vi "Main.vi"() -> ()   [LabVIEW 2020]
uses:
  <vilib>/Utility/NIReport.llb/Create Report.vi
  <vilib>/addons/_office/excel.llb/Excel Get Data.vi
  <vilib>/addons/_office/excel.llb/Excel Get Data ([str]).vi
  <vilib>/Utility/NIReport.llb/NI_report.lvclass
panel:
  in  "文件路径":path
  out "计时器":i32 caption="已用时间(s)" format="%<%H:%M:%S>t"
  in  "过程停止按钮":bool
  in  "复位按钮":bool
  out "结束指示灯":bool
  out "数据导入指示灯":bool
  out "显示屏":string
  in  "抽取按钮":bool
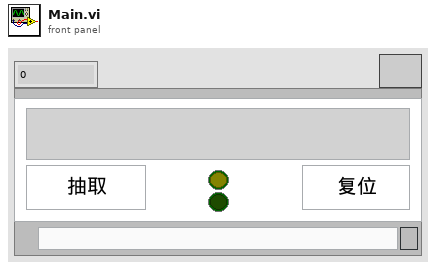
[diagram p1: front panel]
types:
  T1 = enum8{"Enabled", "Disabled", "Disabled and Grayed Out"}
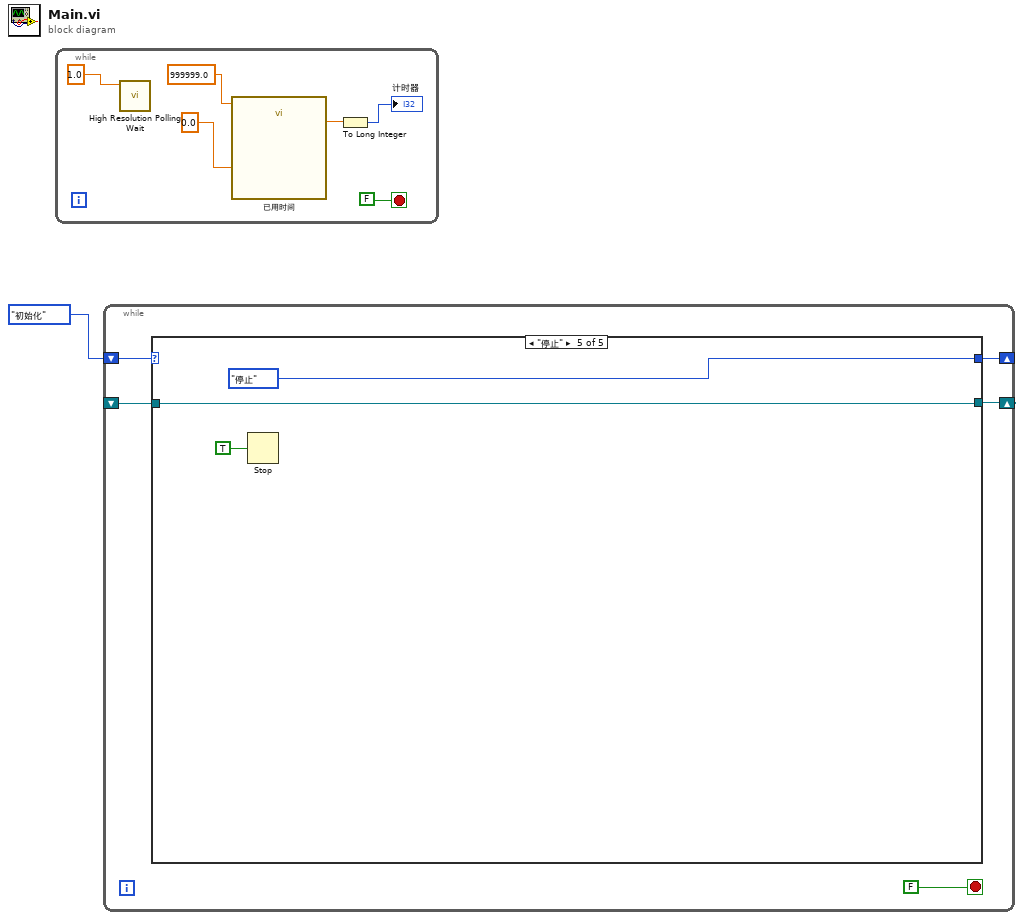
[diagram p0: block diagram]
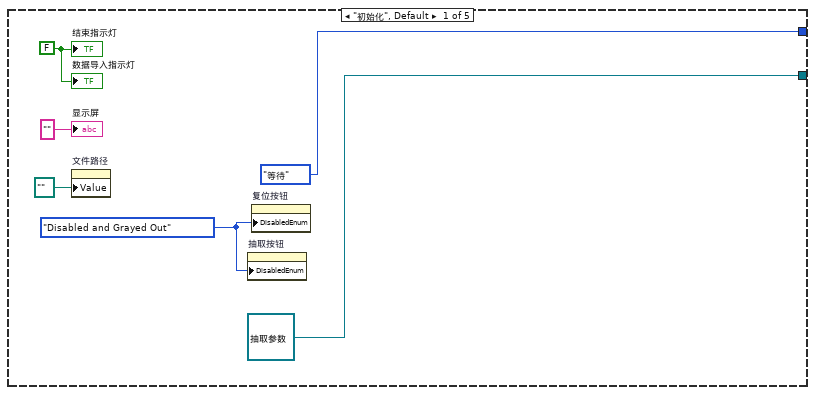
[diagram p2: hidden frame]
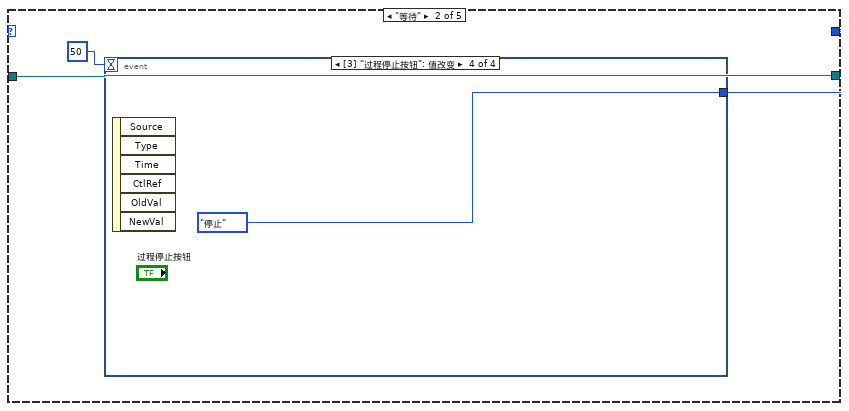
[diagram p3: hidden frame]
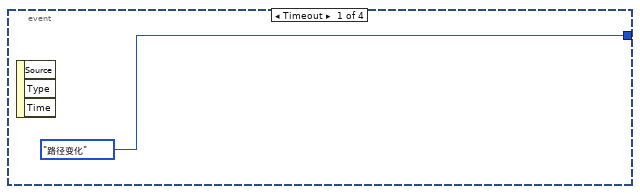
[diagram p4: hidden frame]
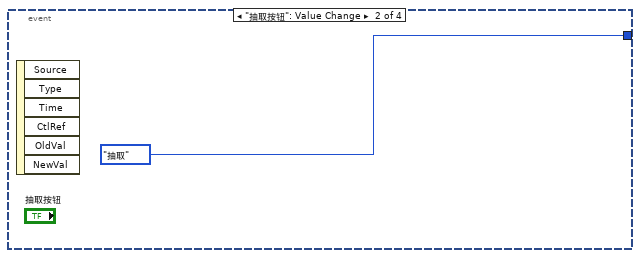
[diagram p5: hidden frame]
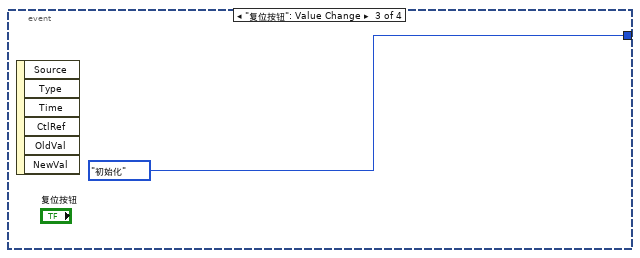
[diagram p6: hidden frame]
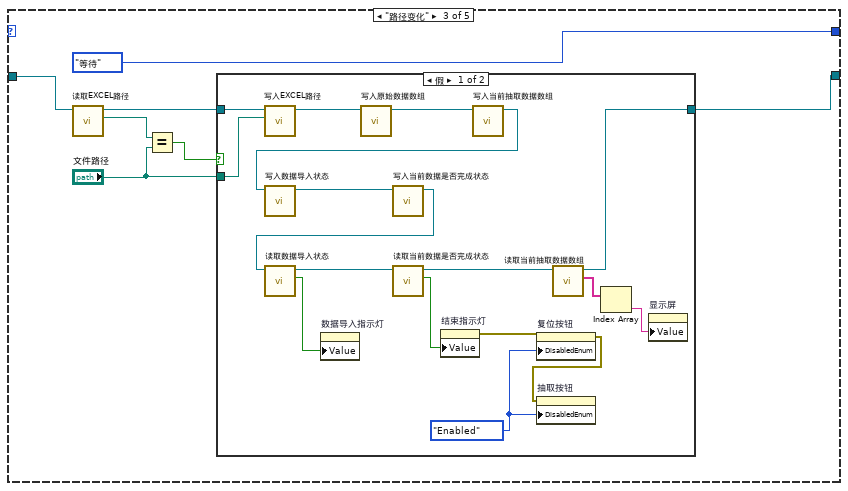
[diagram p7: hidden frame]
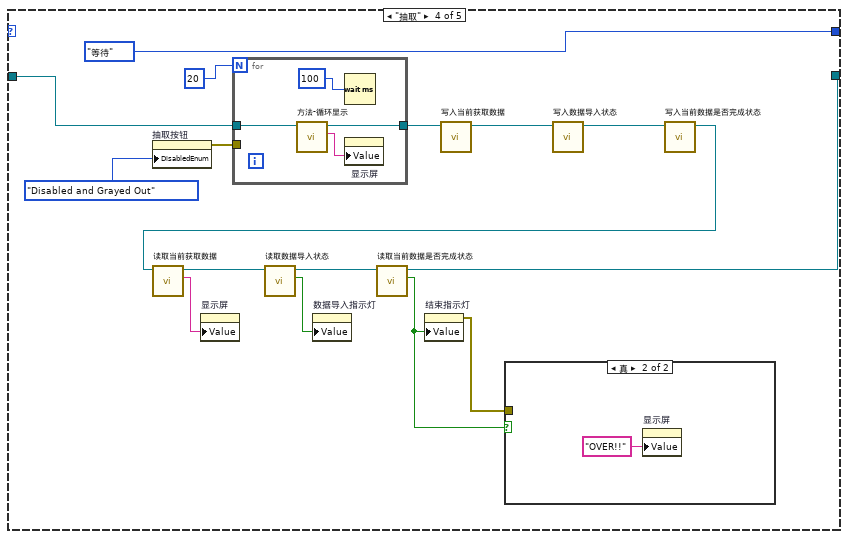
[diagram p9: hidden frame]
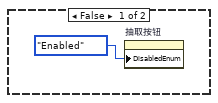
[diagram p10: hidden frame]
diagram:
  n1 = while {
    stop <- FALSE stop-if-true
    n2 = call <vilib>:"High Resolution Polling Wait.vi"("seconds to wait"=1.0) -> ()  [unwired: 10 in, 1 out]
    n3 = call "已用时间"("Time Target (s)"=999999.0, "Set Start Time (s)"=0.0) -> ("Elapsed Time (s)"=w4:dbl)  [unwired: 10 in, 7 out]
    n4 = To Long Integer(number=w4) -> (32bit integer=→"计时器":i32)
  }
  n5 = while {
    shift-right: [w11] -> _
    shift-left: enum16{"初始化", "等待", "路径变化", "抽取", "停止"}."初始化" -> [w12]
    shift-right: [w10] -> _
    shift-left: _ -> [w9]
    stop <- FALSE stop-if-true
    n6 = case shown="\"停止\"" w12 {
      tunnel: [enum16{"初始化", "等待", "路径变化", "抽取", "停止"}."等待" w20 enum16{"初始化", "等待", "路径变化", "抽取", "停止"}."等待" enum16{"初始化", "等待", "路径变化", "抽取", "停止"}."等待" enum16{"初始化", "等待", "路径变化", "抽取", "停止"}."停止"] -> w11
      tunnel: [refnum<class "抽取参数.lvclass"> refnum ("抽取参数.lvclass") w19 w27 w52 w74] -> w10
      tunnel: w9 -> [_ w19 w31 w62 w74]
      frame "初始化", Default {
        w15 = T1."Disabled and Grayed Out" ("禁用")
        w18 = FALSE ("结束指示灯")
        n7 = property on="文件路径" class="Path"("Value"=path "" ("文件路径")) -> ()  [unwired: 2 in, 2 out]
        n8 = property on="抽取按钮" class="Bool"("DisabledEnum"=w15) -> ()  [unwired: 2 in, 2 out]
        n9 = property on="复位按钮" class="Bool"("DisabledEnum"=w15) -> ()  [unwired: 2 in, 2 out]
        "结束指示灯" <- w18
        "数据导入指示灯" <- w18
        "显示屏" <- "" ("显示屏")
      }
      frame "等待" {
        n10 = event shown="[3] \"过程停止按钮\": 值改变" {
          selector: _ -> [_ _ _ _]
          dyn-events: _ -> [_ _ _ _]
          timeout: 50 -> [_ _ _ _]
          tunnel: [enum16{"初始化", "等待", "路径变化", "抽取", "停止"}."路径变化" enum16{"初始化", "等待", "路径变化", "抽取", "停止"}."抽取" enum16{"初始化", "等待", "路径变化", "抽取", "停止"}."初始化" enum16{"初始化", "等待", "路径变化", "抽取", "停止"}."停止"] -> w20
          event Timeout {
            n11 = event-data() -> ()  [unwired: 1 in, 3 out]
          }
          event "抽取按钮": Value Change {
            n12 = event-data() -> ()  [unwired: 1 in, 6 out]
          }
          event "复位按钮": Value Change {
            n13 = event-data() -> ()  [unwired: 1 in, 6 out]
          }
          event "过程停止按钮": Value Change {
            n14 = event-data() -> ()  [unwired: 1 in, 6 out]
          }
        }
      }
      frame "路径变化" {
        n15 = call "读取EXCEL路径.vi"("抽取参数输入"=w31) -> ("EXCEL路径"=w30:path, "抽取参数输出"=w28:refnum<class "抽取参数.lvclass">)  [unwired: 8 in, 1 out]
        n16 = Equal?(x=w30, y="文件路径") -> (x = y?=w29:bool)
        n17 = case shown="假" w29 {
          tunnel: w28 -> [w49 w50]
          tunnel: [w33 w50] -> w27
          tunnel: "文件路径" -> [w48 _]
          frame False {
            w39 = T1."Enabled" ("禁用")
            n18 = call "写入EXCEL路径.vi"("EXCEL路径"=w48, "抽取参数输入"=w49) -> ("抽取参数输出"=w47:refnum<class "抽取参数.lvclass">)  [unwired: 8 in, 1 out]
            n19 = call "写入原始数据数组.vi"("抽取参数输入"=w47) -> ("抽取参数输出"=w46:refnum<class "抽取参数.lvclass">)  [unwired: 9 in, 1 out]
            n20 = call "写入当前抽取数据数组.vi"("抽取参数输入"=w46) -> ("抽取参数输出"=w45:refnum<class "抽取参数.lvclass">)  [unwired: 9 in, 1 out]
            n21 = call "写入数据导入状态.vi"("抽取参数输入"=w45) -> ("抽取参数输出"=w44:refnum<class "抽取参数.lvclass">)  [unwired: 9 in, 1 out]
            n22 = call "写入当前数据是否完成状态.vi"("抽取参数输入"=w44) -> ("抽取参数输出"=w43:refnum<class "抽取参数.lvclass">)  [unwired: 9 in, 1 out]
            n23 = call "读取数据导入状态.vi"("抽取参数输入"=w43) -> ("数据导入状态"=w42:bool, "抽取参数输出"=w41:refnum<class "抽取参数.lvclass">)  [unwired: 8 in, 1 out]
            n24 = property on="数据导入指示灯" class="Bool (严格)"("Value"=w42) -> ()  [unwired: 2 in, 2 out]
            n25 = call "读取当前数据是否完成状态.vi"("抽取参数输入"=w41) -> ("当前数据是否完成状态"=w40:bool, "抽取参数输出"=w36:refnum<class "抽取参数.lvclass">)  [unwired: 8 in, 1 out]
            n26 = property on="结束指示灯" class="Bool (严格)"("Value"=w40) -> (error out=w38:errorcluster)  [unwired: 2 in, 1 out]
            n27 = property on="复位按钮" class="Bool"(error in=w38, "DisabledEnum"=w39) -> (error out=w37:errorcluster)  [unwired: 1 in, 1 out]
            n28 = property on="抽取按钮" class="Bool"(error in=w37, "DisabledEnum"=w39) -> ()  [unwired: 1 in, 2 out]
            n29 = call "读取当前抽取数据数组.vi"("抽取参数输入"=w36) -> ("当前抽取数据数组"=w35:string[], "抽取参数输出"=w33:refnum<class "抽取参数.lvclass">)  [unwired: 8 in, 1 out]
            n30 = Index Array(array=w35) -> (element=w34:string)  [unwired: 1 in]
            n31 = property on="显示屏" class="Str"("Value"=w34) -> ()  [unwired: 2 in, 2 out]
          }
          frame True {
          }
        }
      }
      frame "抽取" {
        n32 = property on="抽取按钮" class="Bool"("DisabledEnum"=T1."Disabled and Grayed Out" ("禁用")) -> (error out=w63:errorcluster)  [unwired: 2 in, 1 out]
        n33 = for {
          N: 20 -> [_]
          tunnel: w63 -> [_]
          tunnel: w62 -> [w71]
          tunnel: [w70] -> w61
          n34 = call "方法-循环显示.vi"("抽取参数 输入"=w71) -> ("循环显示元素"=w72:string, "抽取参数 输出"=w70:refnum<class "抽取参数.lvclass">)  [unwired: 8 in, 1 out]
          n35 = Wait (ms)(milliseconds to wait=u32 100) -> ()  [unwired: 1 out]
          n36 = property on="显示屏" class="Str"("Value"=w72) -> ()  [unwired: 2 in, 2 out]
        }
        n37 = call "写入当前获取数据.vi"("抽取参数输入"=w61) -> ("抽取参数输出"=w60:refnum<class "抽取参数.lvclass">)  [unwired: 9 in, 1 out]
        n38 = call "写入数据导入状态.vi"("抽取参数输入"=w60) -> ("抽取参数输出"=w59:refnum<class "抽取参数.lvclass">)  [unwired: 9 in, 1 out]
        n39 = call "写入当前数据是否完成状态.vi"("抽取参数输入"=w59) -> ("抽取参数输出"=w58:refnum<class "抽取参数.lvclass">)  [unwired: 9 in, 1 out]
        n40 = call "读取当前获取数据.vi"("抽取参数输入"=w58) -> ("当前获取数据"=w55:string, "抽取参数输出"=w57:refnum<class "抽取参数.lvclass">)  [unwired: 8 in, 1 out]
        n41 = property on="显示屏" class="Str"("Value"=w55) -> ()  [unwired: 2 in, 2 out]
        n42 = call "读取数据导入状态.vi"("抽取参数输入"=w57) -> ("数据导入状态"=w54:bool, "抽取参数输出"=w56:refnum<class "抽取参数.lvclass">)  [unwired: 8 in, 1 out]
        n43 = property on="数据导入指示灯" class="Bool (严格)"("Value"=w54) -> ()  [unwired: 2 in, 2 out]
        n44 = call "读取当前数据是否完成状态.vi"("抽取参数输入"=w56) -> ("当前数据是否完成状态"=w53:bool, "抽取参数输出"=w52:refnum<class "抽取参数.lvclass">)  [unwired: 8 in, 1 out]
        n45 = property on="结束指示灯" class="Bool (严格)"("Value"=w53) -> (error out=w51:errorcluster)  [unwired: 2 in, 1 out]
        n46 = case shown="真" w53 {
          tunnel: w51 -> [_ _]
          frame False {
            n47 = property on="抽取按钮" class="Bool"("DisabledEnum"=T1."Enabled" ("禁用")) -> ()  [unwired: 2 in, 2 out]
          }
          frame True {
            n48 = property on="显示屏" class="Str"("Value"="OVER!!" ("显示屏")) -> ()  [unwired: 2 in, 2 out]
          }
        }
      }
      frame "停止" {
        n49 = Stop(stop? (T)=TRUE ("停止？(T)")) -> ()
      }
    }
  }
